vi "ToString.vi"(8 "error in (no error)":errorcluster, 11 "ErrorCode in":refnum<class "ErrorCode.lvclass">) -> (0 "error out":errorcluster, 2 "String":string, 3 "ErrorCode out":refnum<class "ErrorCode.lvclass">)   [LabVIEW 2017, in "Transparent Assertions.lvlib" / "Constraints.lvlib" / "ErrorCode.lvclass"]
doc: "Returns a string representation of the object."
uses:
  ErrorCode.lvclass
  ErrorCode.lvclass/ErrorCode.ctl
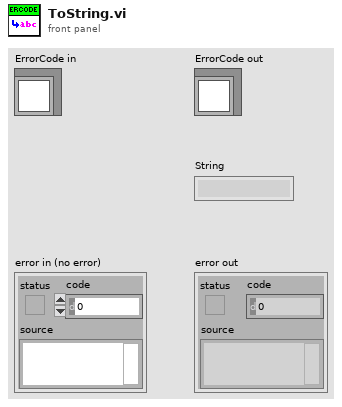
[diagram p1: front panel]
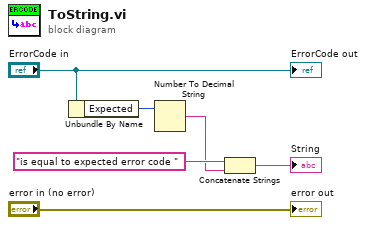
[diagram p0: block diagram]
diagram:
  n1 = Unbundle By Name("ErrorCode in") -> ("Expected"=w2:i32)
  n2 = Number To Decimal String(number=w2) -> (decimal integer string=w1:string)  [unwired: 1 in]
  n3 = Concatenate Strings("is equal to expected error code " ("String"), w1) -> (→"String":string)
  "error out" <- "error in (no error)"
  "ErrorCode out" <- "ErrorCode in"
